vi "Replace Configuration Table By ID.vi"   [LabVIEW 2017]
doc: "Palette helper grouping the two Replace Configuration Table By ID instances, which replace a single row or an array of rows selected by their ID column."
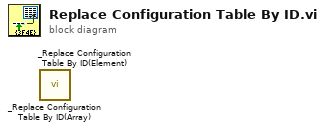
[diagram p0: block diagram]
diagram:
  n1 = call "_Replace Configuration Table By ID(Array).vi"() -> ()  [unwired: 10 in, 2 out]
  n2 = call "_Replace Configuration Table By ID(Element).vi"() -> ()  [unwired: 10 in, 2 out]
